vi "Configure Button from File.vi"(0 "Display State In":T1={"Header"="", "Label[]"=[], "DisableButtonsLUT"=variant(string[] []), "Menu Config"=variant}, 5 "Configuration Path":path, 9 "Container State":T2, 11 "error in (no error)":errorcluster) -> (4 "Display State Out":T1={"Header"="", "Label[]"=[], "DisableButtonsLUT"=variant(string[] []), "Menu Config"=variant}, 6 "Ok?":bool, 8 "MenuConfig":variant, 15 "error out":errorcluster)   [LabVIEW 2019, in "Menu Button.xctl"]
doc: "JSMA Module Template - Top Level UI 0.2.0.4\nRob Humfeld - Jet Engineering\nCopyright (c) 2019, Jet Engineering"
uses:
  Menu Button.xctl
  <vilib>/_xctls/Container State.ctl
  State 1.ctl
  <vilib>/_xctls/XControlSupport.lvlib
panel:
  # "Add Controls & Indicators that form the parameters of the method here. Hook them to the connector pane. Do not delete the controls & indicators that are already hooked to the connector pane.\n \nTo setup the parameters  for this method, right click on this item in the Project Tree & select \"Configure Method...\"."
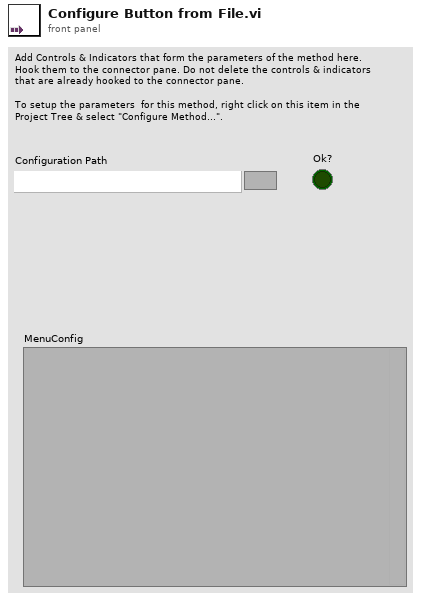
[diagram p1: front panel]
types:
  T1 = typedef "Menu Button.xctl/State 1.ctl" = cluster{"Header":string, "Label[]":string[], "DisableButtonsLUT":variant, "Menu Config":variant}
  T2 = typedef "XControlSupport.lvlib/Container State.ctl" = cluster{"Indicator?":bool, "Run Mode?":bool, " Refnum":refnum<vi>}
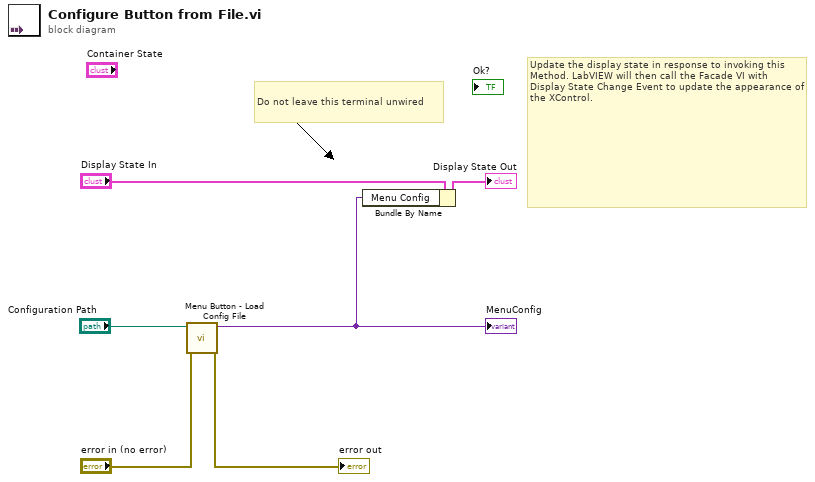
[diagram p0: block diagram]
diagram:
  # "Do not leave this terminal unwired"
  # "Update the display state in response to invoking this Method. LabVIEW will then call the Facade VI with Display State Change Event to update the appearance of the XControl."
  n1 = call "Menu Button - Load Config File.vi"("error in (no error)"="error in (no error)", "Path"="Configuration Path") -> ("error out"=→"error out":errorcluster, "MenuConfig"=w1:variant)  [unwired: 6 in, 2 out]
  "MenuConfig" <- w1
  n2 = Bundle By Name(cluster="Display State In", "Menu Config"=w1) -> (→"Display State Out":T1)
